vi "SaveAlarms.vi"(8 "error in (no error)":errorcluster, 9 "data":T9, 10 "data event in":T1) -> (0 "error out":errorcluster, 3 "data event out":T1)   [LabVIEW 2017, in "IrDataEventCreator.lvlib"]
uses:
  <vilib>/addons/InsightCM/Devices/Shared/Ir/IrDataEventCreator/IrDataEventCreator.lvlib
  <vilib>/addons/InsightCM/Devices/Shared/Common/DataFlow/controls/Data.ctl
  <vilib>/addons/InsightCM/Utilities/DataAccessors/controls/wfmSGL_DVR.ctl
  <vilib>/addons/PointValueMap/controls/PointMap.ctl
  <vilib>/addons/InsightCM/Devices/Shared/Common/DataFlow/controls/Type.ctl
  <vilib>/addons/InsightCM/Devices/Shared/Common/DataEvent/controls/Event.ctl
  <vilib>/addons/InsightCM/MessageBus/Base/controls/DataEvent.ctl
  <vilib>/addons/InsightCM/MessageBus/Base/controls/KeyValuePair.ctl
  <vilib>/addons/InsightCM/Devices/Shared/Common/DataEvent/controls/DataSet.ctl
  <vilib>/addons/InsightCM/MessageBus/Base/controls/DataSetMetadata.ctl
  <vilib>/addons/InsightCM/MessageBus/Base/controls/TrendPoint.ctl
  <vilib>/addons/InsightCM/MessageBus/Base/controls/TrendAlarmUpdate.ctl
  <vilib>/addons/InsightCM/MessageBus/Base/controls/TrendAlarmTransition.ctl
  <vilib>/addons/PointValueMap/subVIs/Point_Read_variant.vi
  <vilib>/addons/PointValueMap/PointValueMap.lvlib
  <vilib>/addons/InsightCM/Devices/Shared/Common/DataFlow/DataFlow.lvlib
  <vilib>/addons/InsightCM/Devices/Shared/Common/DataEvent/DataEvent.lvlib
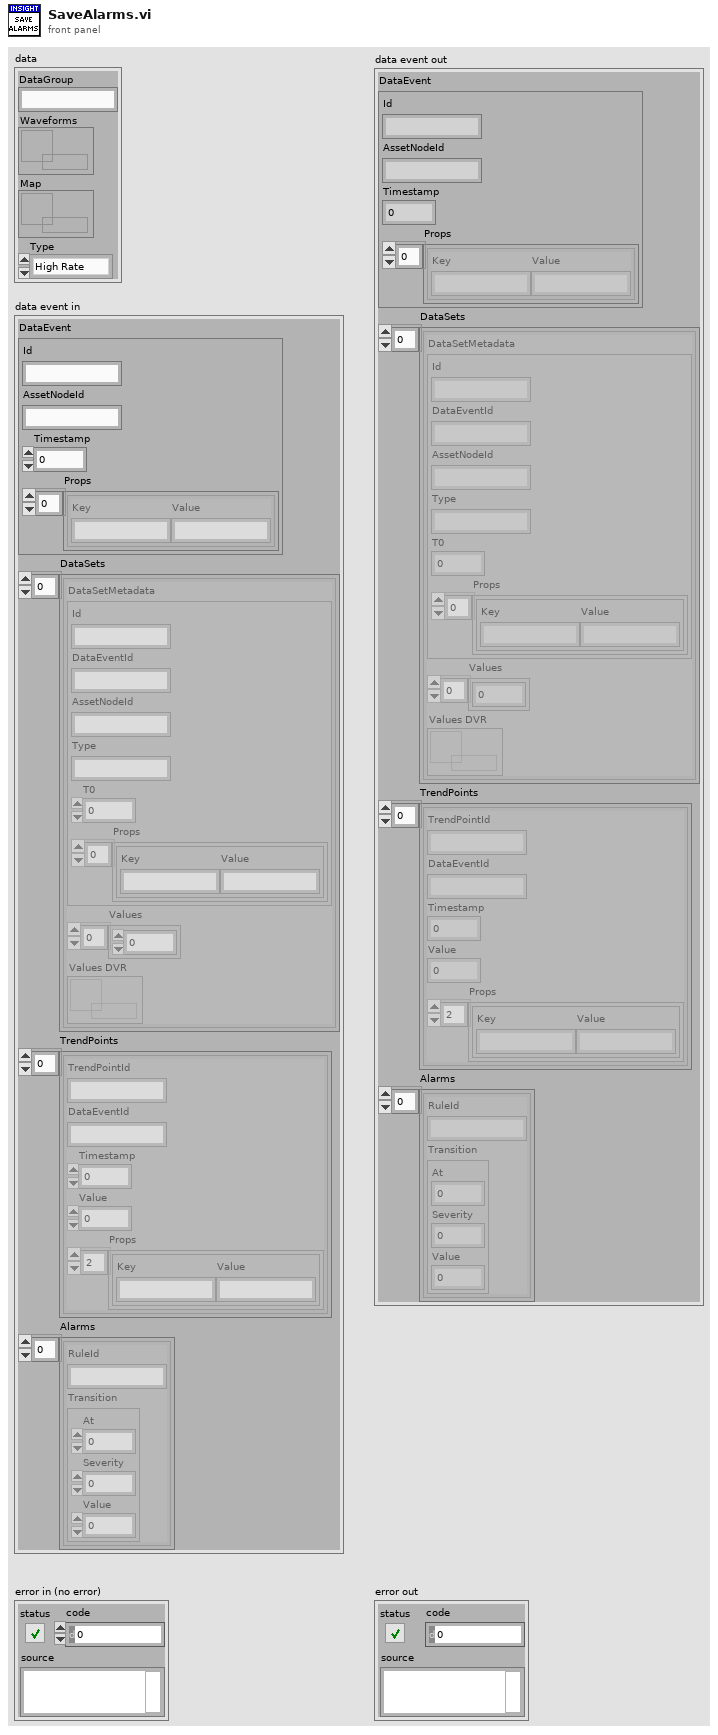
[diagram p1: front panel]
types:
  T1 = typedef "DataEvent.lvlib/Event.ctl" = cluster{"DataEvent":T2, "DataSets":T4[], "TrendPoints":T6[], "Alarms":T7[]}
  T2 = typedef "DataEvent.ctl" = cluster{"Id":string, "AssetNodeId":string, "Timestamp":i64, "Props":T3[]}
  T3 = typedef "KeyValuePair.ctl" = cluster{"Key":string, "Value":string}
  T4 = typedef "DataEvent.lvlib/DataSet.ctl" = cluster{"DataSetMetadata":T5, "Values":sgl[], "Values DVR":refnum<data-value>}
  T5 = typedef "DataSetMetadata.ctl" = cluster{"Id":string, "DataEventId":string, "AssetNodeId":string, "Type":string, "T0":i64, "Props":T3[]}
  T6 = typedef "TrendPoint.ctl" = cluster{"TrendPointId":string, "DataEventId":string, "Timestamp":i64, "Value":dbl, "Props":T3[]}
  T7 = typedef "TrendAlarmUpdate.ctl" = cluster{"RuleId":string, "Transition":T8}
  T8 = typedef "TrendAlarmTransition.ctl" = cluster{"At":i64, "Severity":i32, "Value":dbl}
  T9 = typedef "DataFlow.lvlib/Data.ctl" = cluster{"DataGroup":string, "Waveforms":T10, "Map":T11, "Type":T12}
  T10 = typedef "wfmSGL_DVR.ctl" = refnum<data-value>
  T11 = typedef "PointValueMap.lvlib/PointMap.ctl" = refnum<data-value>
  T12 = typedef "DataFlow.lvlib/Type.ctl" = enum16{"High Rate", "Low Rate", "Burst Mode"}
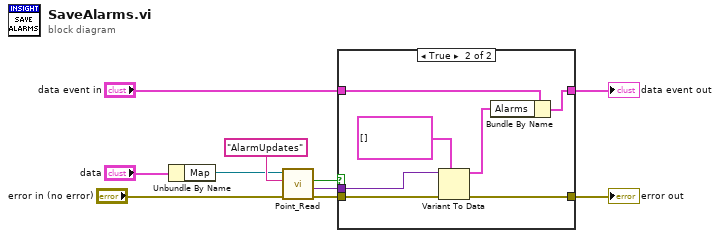
[diagram p0: block diagram]
diagram:
  n1 = Unbundle By Name("data") -> ("Map"=w9:T11)
  n2 = call-poly <vilib>:"Point_Read.vi"("Error In"="error in (no error)", "Tag"="AlarmUpdates", "Map"=w9) -> ("Error Out"=w5:errorcluster, "Value"=w1:variant, "Found?"=w4:bool)  [unwired: 3 in, 3 out]
  n3 = case shown="True" w4 {
    tunnel: [w11 w15] -> w6
    tunnel: w5 -> [w11 w16]
    tunnel: "data event in" -> [w12 w19]
    tunnel: [w12 w18] -> w2
    tunnel: w1 -> [_ w14]
    frame False {
    }
    frame True {
      n4 = Variant To Data(error in=w16, type=T7[] [], Variant=w14) -> (data=w13:T7[], error out=w15:errorcluster)
      n5 = Bundle By Name(cluster=w19, "Alarms"=w13) -> (w18:T1)
    }
  }
  "error out" <- w6
  "data event out" <- w2
